vi "testing.vi"() -> ()   [LabVIEW 2017]
panel:
  out "Both":bool
  in  "R-U":bool
  in  "L-U":bool
  in  "L-d":bool
  in  "R-d":bool
  in  "left":bool
  in  "right":bool
  in  "down":bool
  in  "up":bool
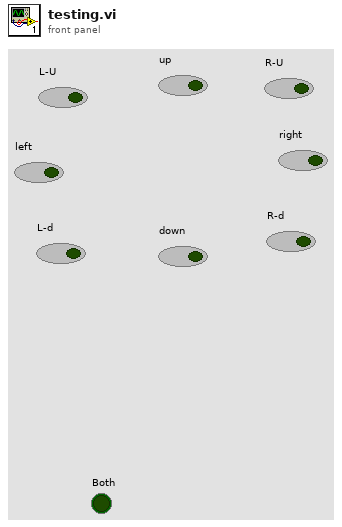
[diagram p1: front panel]
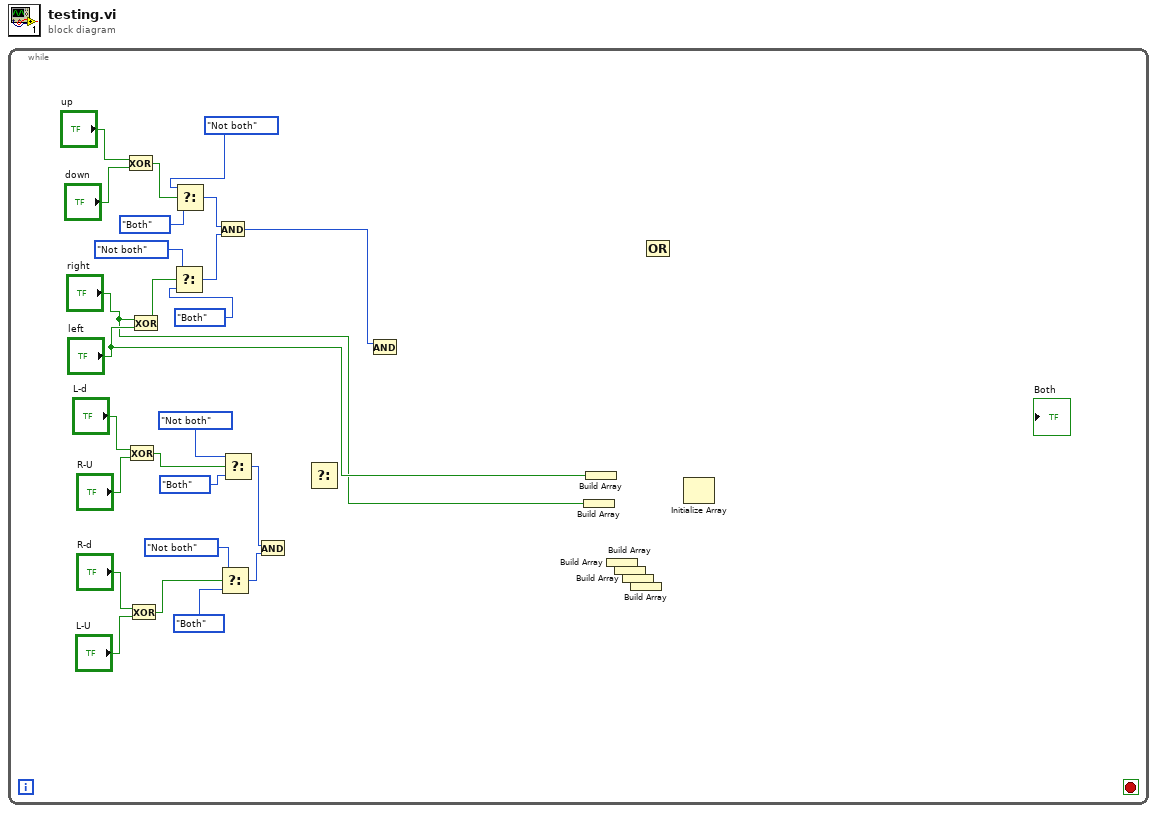
[diagram p0: block diagram]
diagram:
  n1 = while {
    stop <- _ stop-if-true
    n2 = Exclusive Or(1:"down", 2:"up") -> (0:w19:bool)
    n3 = Exclusive Or(1:"R-U", 2:"L-d") -> (0:w9:bool)
    n4 = Exclusive Or(1:"L-U", 2:"R-d") -> (0:w8:bool)
    n5 = Exclusive Or(1:"left", 2:"right") -> (0:w18:bool)
    n6 = Select(t=enum16{"Not both", "Both"}."Not both", s=w18, f=enum16{"Not both", "Both"}."Both") -> (s? t:f=w17:enum16{"Not both", "Both"})
    n7 = Select(t=enum16{"Not both", "Both"}."Not both", s=w19, f=enum16{"Not both", "Both"}."Both") -> (s? t:f=w16:enum16{"Not both", "Both"})
    n8 = And(x=w16, y=w17) -> (x .and. y?=w3:i32)
    n9 = Select(t=enum16{"Not both", "Both"}."Not both", s=w8, f=enum16{"Not both", "Both"}."Both") -> (s? t:f=w5:enum16{"Not both", "Both"})
    n10 = Select(t=enum16{"Not both", "Both"}."Not both", s=w9, f=enum16{"Not both", "Both"}."Both") -> (s? t:f=w4:enum16{"Not both", "Both"})
    n11 = And(x=w4, y=w5) -> ()  [unwired: 1 out]
    n12 = Select() -> ()  [unwired: 3 in, 1 out]
    n13 = And(x=w3) -> ()  [unwired: 1 in, 1 out]
    n14 = Build Array("right") -> ()  [unwired: 1 out]
    n15 = Build Array("left") -> ()  [unwired: 1 out]
    n16 = Build Array() -> ()  [unwired: 1 in, 1 out]
    n17 = Build Array() -> ()  [unwired: 1 in, 1 out]
    n18 = Build Array() -> ()  [unwired: 1 in, 1 out]
    n19 = Build Array() -> ()  [unwired: 1 in, 1 out]
    n20 = Compound Arithmetic op=OR() -> ()  [unwired: 2 in, 1 out]
    n21 = Initialize Array() -> ()  [unwired: 2 in, 1 out]
  }
